vi "tierra.vi"() -> ()   [LabVIEW 2016]
uses:
  <vilib>/picture/3D Picture Control/Object/Create Object (drawable).vi
  <vilib>/picture/3D Picture Control/Helpers/Apply Texture (no reference).vi
  <vilib>/picture/3D Picture Control/Object/Add Object (no reference).vi
  <vilib>/picture/3D Picture Control/NI_3D Picture Control.lvlib
panel:
  in  "path to JPEG file":path
  out "3D Picture":refnum<vi>(3d-picture)
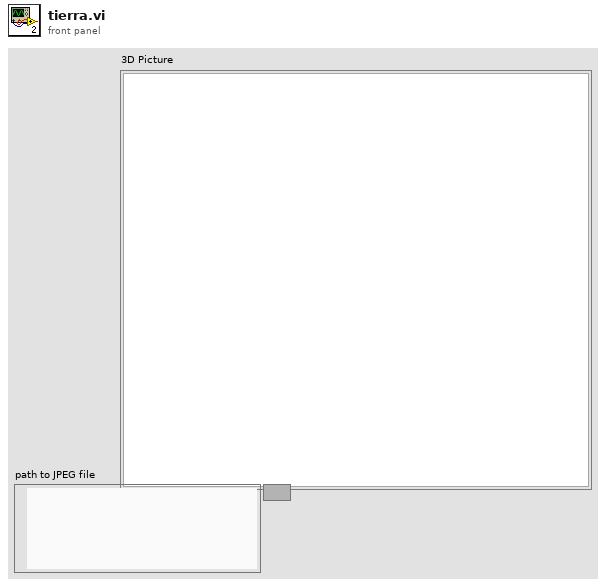
[diagram p1: front panel]
types:
  T1 = cluster{"Red":sgl, "Green":sgl, "Blue":sgl, "Alpha":sgl}
  T2 = typedef "imagedata.ctl" = cluster{"image type":i32, "image depth":i32, "image":u8[], "mask":u8[], "colors":u32[], "Rectangle":cluster{"left":i16, "top":i16, "right":i16, "bottom":i16}}
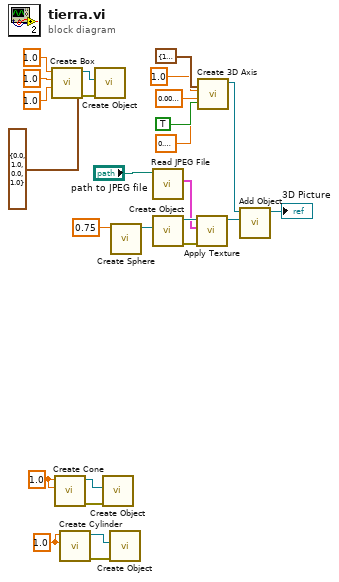
[diagram p0: block diagram]
diagram:
  w10 = sgl 1.0 ("Radius")
  w13 = sgl 1.0 ("Height")
  n1 = call <vilib>:"Create Box.vi"("Color"=T1 {"Red"=0.0, "Green"=1.0, "Blue"=0.0, "Alpha"=1.0}, "Length Z"=sgl 1.0, "Length Y"=sgl 1.0, "Length X"=sgl 1.0) -> ("error out"=w17:errorcluster, "New Box Refnum"=w16:refnum<vi>)  [unwired: 6 in]
  n2 = call <vilib>:"Create Cone.vi"("Radius"=w13, "Height"=w13) -> ("error out"=w11:errorcluster, "New Cone Refnum"=w12:refnum<vi>)  [unwired: 8 in]
  n3 = call <vilib>:"Create Cylinder.vi"("Radius"=w10, "Height"=w10) -> ("error out"=w9:errorcluster, "New Cylinder Refnum"=w8:refnum<vi>)  [unwired: 8 in]
  n4 = call-poly <vilib>:"Create Object.vi"("error in (no error)"=w17, "Geometry"=w16) -> ()  [unwired: 8 in, 2 out]
  n5 = call-poly <vilib>:"Create Object.vi"("error in (no error)"=w11, "Geometry"=w12) -> ()  [unwired: 8 in, 2 out]
  n6 = call-poly <vilib>:"Create Object.vi"("error in (no error)"=w9, "Geometry"=w8) -> ()  [unwired: 8 in, 2 out]
  n7 = call <vilib>:"Create Sphere.vi"("Radius"=sgl 0.75) -> ("New Sphere Refnum"=w14:refnum<vi>)  [unwired: 9 in, 1 out]
  n8 = call <vilib>:"Read JPEG File.vi"("path to JPEG file"="path to JPEG file") -> ("image data"=w4:T2)  [unwired: 8 in, 2 out]
  n9 = call-poly <vilib>:"Create Object.vi"("Geometry"=w14) -> ("error out"=w6:errorcluster, "Scene:New Object"=w5:refnum<vi>)  [unwired: 9 in]
  n10 = call-poly <vilib>:"Apply Texture.vi"("error in (no error)"=w6, "Image Data"=w4, "Scene Object In"=w5) -> ("Scene Object Out"=w1:refnum<vi>)  [unwired: 7 in, 1 out]
  n11 = call <vilib>:"Create 3D Axis.vi"("Character Size"=sgl 0.2, "Axis label?"=TRUE, "Color"=T1 {"Red"=1.0, "Green"=1.0, "Blue"=1.0, "Alpha"=1.0}, "Radius"=sgl 0.01, "Length"=sgl 1.0) -> ("New Object Refnum"=w7:refnum<vi>)  [unwired: 5 in, 1 out]
  n12 = call-poly <vilib>:"Add Object.vi"("New Object In"=w1, "Scene Object In"=w7) -> ("Scene Object Out"=→"3D Picture":refnum<vi>)  [unwired: 8 in, 1 out]
